vi "thres_conf_ASIC.vi"(6 "threshold":u32, 7 "Ring":u16(ring)=5 items=["Channel 0", "Channel 1", "Channel 2", "Channel 3", "Channel 4", "Channel 5", "Channel 6"], 8 "error out 3":errorcluster, 10 "Id in":i32, 11 "connection ID":refnum<k5>) -> (0 "error out 2":errorcluster, 2 "data read value":u32, 3 "connection ID out":refnum<k5>, 5 "Id out":i32=72)   [LabVIEW 2009]
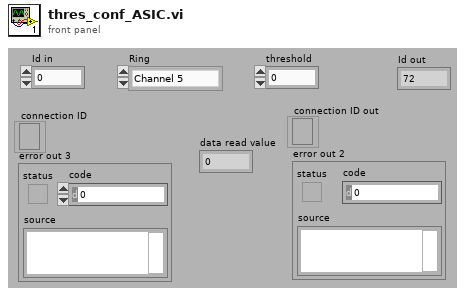
[diagram p1: front panel]
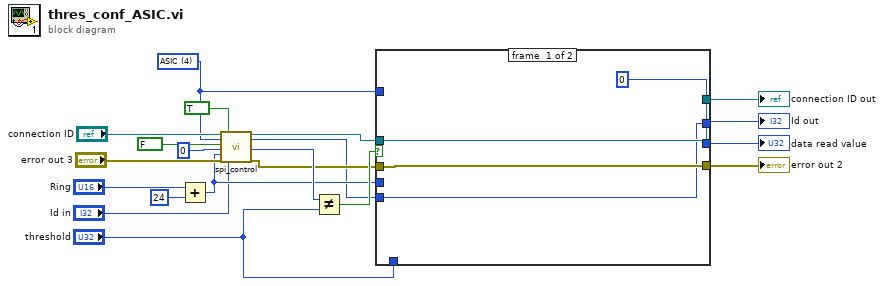
[diagram p0: block diagram]
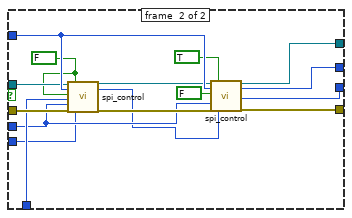
[diagram p2: hidden frame]
diagram:
  w16 = u16 4 items=["Attenuation", "Clipping", "Enable channel", "Delay line", "ASIC"] ("Device")
  n1 = Add(x="Ring", y=u16 24) -> (x+y=w7:u16)
  n2 = call "spi_control.vi"("connection ID"="connection ID", "Device"=w16, "Read/#write"=FALSE, "Data"=0, "Register or channel"=w7, "error out 3"="error out 3", "Read physical"=TRUE, "Id in"="Id in") -> ("connection ID out"=w15:refnum<k5>, "Id out"=w6:i32, "data read value"=w18:u32, "error out 2"=w14:errorcluster)  [unwired: 4 in, 4 out]
  n3 = Not Equal?(x=w18, y="threshold") -> (x != y?=w17:bool)
  n4 = case shown="True" w17 {
    tunnel: w16 -> [_ w40]
    tunnel: w15 -> [w24 w38]
    tunnel: w14 -> [w23 w37]
    tunnel: "threshold" -> [_ w35]
    tunnel: w7 -> [_ w34]
    tunnel: w6 -> [w22 w29]
    tunnel: [w23 w28] -> w5
    tunnel: [w24 w27] -> w4
    tunnel: [0 ("Id out") w26] -> w3
    tunnel: [w22 w25] -> w2
    frame #0 {
    }
    frame #1 {
      w31 = FALSE ("Read physical")
      n5 = call "spi_control.vi"("connection ID"=w38, "Device"=w40, "Read/#write"=w31, "Data"=w35, "Register or channel"=w34, "error out 3"=w37, "Read physical"=w31, "Id in"=w29) -> ("connection ID out"=w39:refnum<k5>, "Id out"=w30:i32, "error out 2"=w36:errorcluster)  [unwired: 4 in, 5 out]
      n6 = call "spi_control.vi"("connection ID"=w39, "Device"=w40, "Read/#write"=FALSE, "Register or channel"=w34, "error out 3"=w36, "Read physical"=TRUE, "Id in"=w30) -> ("connection ID out"=w27:refnum<k5>, "Id out"=w25:i32, "data read value"=w26:u32, "error out 2"=w28:errorcluster)  [unwired: 5 in, 4 out]
    }
  }
  "connection ID out" <- w4
  "error out 2" <- w5
  "Id out" <- w2
  "data read value" <- w3
